vi "read_acknowledge.vi"(8 "error in (no error)":errorcluster, 11 "VISA resource name":refnum<visa-resource-name>) -> (0 "error out":errorcluster, 2 "protocol version":string, 3 "VISA resource name out":refnum<visa-resource-name>)   [LabVIEW 2018]
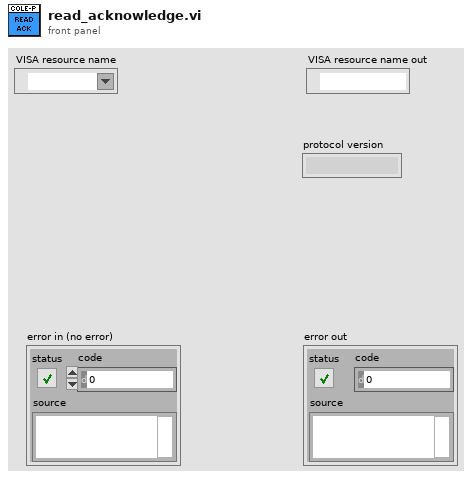
[diagram p1: front panel]
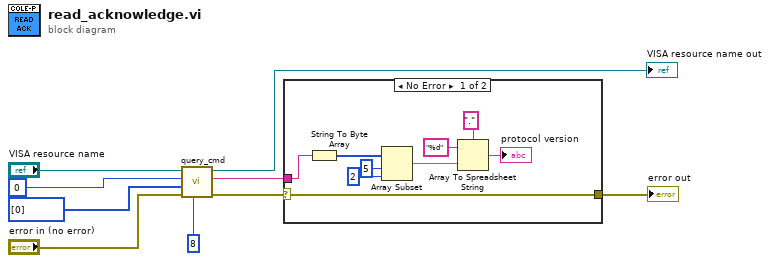
[diagram p0: block diagram]
diagram:
  n1 = call "query_cmd.vi"("Number of bytes in response"=u32 8, "error in (no error)"="error in (no error)", "Data bytes"=u8[] [0], "Command byte"=u8 0, "VISA resource name"="VISA resource name") -> ("error out"=w2:errorcluster, "Response"=w3:string, "VISA resource name out"=→"VISA resource name out":refnum<visa-resource-name>)  [unwired: 4 in]
  n2 = case shown="No Error" w2 {
    selector: w2 -> [w18 w19]
    tunnel: w3 -> [w17 _]
    tunnel: [w18 w19] -> w1
    frame No Error {
      n3 = String To Byte Array(string=w17) -> (unsigned byte array=w16:u8[])
      n4 = Array Subset(array=w16, index=5, length=2) -> (w13:u8[])
      n5 = Array To Spreadsheet String(delimiter (Tab)=".", array=w13, 3:"%d" ("format string")) -> (spreadsheet string=→"protocol version":string)
    }
    frame Error {
    }
  }
  "error out" <- w1
